vi "niFPGA 32-Bit Cast Emit Code.vi"(0 "Emit Code Info In":refnum<class "EmitCode(DiagramComponent).lvclass">, 11 "error in (no error)":errorcluster) -> (4 "Emit Code Info Out":refnum<class "EmitCode(DiagramComponent).lvclass">, 15 "error out":errorcluster)   [LabVIEW 2017]
uses:
  <vilib>/rvi/ClientSDK/Core/ModuleGeneration/ClassModGen/EmitCode(DiagramComponent)/EmitCode(DiagramComponent).lvclass
  e:/penguin/lvdist/win32/export/17.0/17.0.1f1/dist/vi.lib/rvi/ClientSDK/Core/ModuleGeneration/ClassModGen/ModGen/ModGen.lvclass
  e:/penguin/lvdist/win32/export/17.0/17.0.1f1/dist/vi.lib/rvi/ClientSDK/Core/ModuleGeneration/ClassModGen/EmitCode/EmitCode.lvclass
  <vilib>/rvi/ClientSDK/Core/ModuleGeneration/InstantiationUtility/Public/nirviInstantiatedPortSpec.ctl
  <vilib>/rvi/ClientSDK/Core/ModuleGeneration/InstantiationUtility/Public/nirviInstantiatedGenericSpec.ctl
  <vilib>/rvi/ClientSDK/Core/ModuleGeneration/ClassModGen/ModGen/ModGen.lvclass
  <vilib>/rvi/ClientSDK/Core/ModuleGeneration/ClassModGen/EmitCode/EmitCode.lvclass
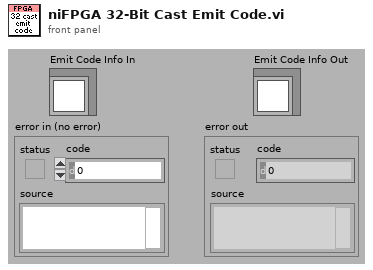
[diagram p1: front panel]
types:
  T1 = typedef "nirviInstantiatedGenericSpec.ctl" = cluster{"Static Generic Connection":string, "Generic Value If Unconnected":string, "Generic Name From Backend":string, "Pre Connection Addition":string, "Post Connection Addition":string}
  T2 = typedef "nirviInstantiatedPortSpec.ctl" = cluster{"Port Name From Backend":string, "Static Port Connection":string, "Post Signal Addition":string, "Pre Signal Addition":string, "Value If Unwired":string, "TxtToReplaceWithActualSig":string}
  T3 = cluster{"PortName":string, "PortConnection":string, "isConstant":bool, "PortWidth":i32, "Direction":enum32{"", "MOD_PORT_OUT", "MOD_PORT_IN", "MOD_PORT_INOUT"}, "Representation":enum32{"", "MOD_SIG_SIGN", "MOD_SIG_UNSIGN", "MOD_SIG_FLOAT"}, "Sig type":enum32{"", "MOD_SIG_BIT", "MOD_SIG_VECT", "MOD_SIG_ARRAY"}, "NumDimensions":i32, "DimensionSizes":i32[], "Element Width":i32, "Generic Name":string}[]
  T4 = typedef "niFpgaGeneric.ctl" = cluster{"Generic Name":string, "Port Type":string, "String Value":string, "Int Value":i64}
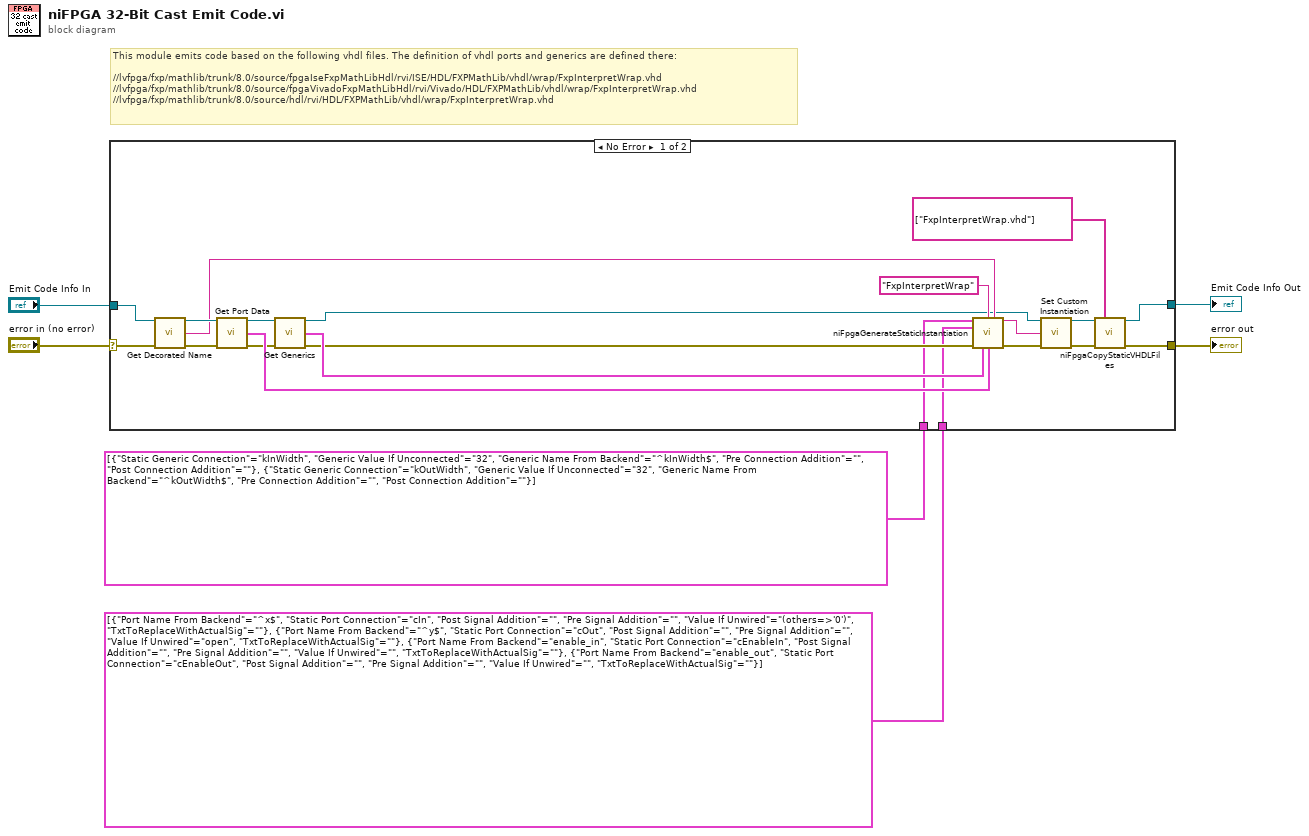
[diagram p0: block diagram]
diagram:
  # "This module emits code based on the following vhdl files. The definition of vhdl ports and generics are defined there:\n\n//lvfpga/fxp/mathlib/trunk/8.0/source/fpgaIseFxpMathLibHdl/rvi/ISE/HDL/FXPMathLib/vhdl/wrap/FxpInterpretWrap.vhd\n//lvfpga/fxp/mathlib/trunk/8.0/source/fpgaVivadoFxpMathLibHdl/rvi/Vivado/HDL/FXPMathLib/vhdl/wrap/FxpInterpretWrap.vhd\n//lvfpga/fxp/mathlib/trunk/8.0/source/hdl/rvi/HDL/FXPMathLib/vhdl/wrap/FxpInterpretWrap.vhd"
  n1 = case shown="No Error" "error in (no error)" {
    selector: "error in (no error)" -> [w16 w28]
    tunnel: "Emit Code Info In" -> [w17 w29]
    tunnel: [w11 w28] -> w5
    tunnel: [w9 w29] -> w4
    tunnel: T2[] [{"Port Name From Backend"="^x$", "Static Port Connection"="cIn", "Post Signal Addition"="", "Pre Signal Addition"="", "Value If Unwired"="(others=>'0')", "TxtToReplaceWithActualSig"=""}, {"Port Name From Backend"="^y$", "Static Port Connection"="cOut", "Post Signal Addition"="", "Pre Signal Addition"="", "Value If Unwired"="open", "TxtToReplaceWithActualSig"=""}, {"Port Name From Backend"="enable_in", "Static Port Connection"="cEnableIn", "Post Signal Addition"="", "Pre Signal Addition"="", "Value If Unwired"="", "TxtToReplaceWithActualSig"=""}, {"Port Name From Backend"="enable_out", "Static Port Connection"="cEnableOut", "Post Signal Addition"="", "Pre Signal Addition"="", "Value If Unwired"="", "TxtToReplaceWithActualSig"=""}] ("Static Ports") -> [w13 _]
    tunnel: T1[] [{"Static Generic Connection"="kInWidth", "Generic Value If Unconnected"="32", "Generic Name From Backend"="^kInWidth$", "Pre Connection Addition"="", "Post Connection Addition"=""}, {"Static Generic Connection"="kOutWidth", "Generic Value If Unconnected"="32", "Generic Name From Backend"="^kOutWidth$", "Pre Connection Addition"="", "Post Connection Addition"=""}] -> [w7 _]
    frame No Error {
      n2 = call <vilib>:"Get Decorated Name.vi"("ModGen in"=w17, "error in (no error)"=w16) -> ("ModGen out"=w24:refnum<class "EmitCode(DiagramComponent).lvclass">, "Decorated Name"=w22:string, "error out"=w23:errorcluster)  [unwired: 11 in]
      n3 = call <vilib>:"Get Port Data.vi"("CodeGenInfo(Resource) in"=w24, "error in (no error)"=w23) -> ("CodeGenInfo(Resource) out"=w19:refnum<class "EmitCode(DiagramComponent).lvclass">, "Port Data"=w26:T3, "error out"=w20:errorcluster)  [unwired: 11 in]
      n4 = call <vilib>:"Get Generics.vi"("ModGenInfo in"=w19, "error in (no error)"=w20) -> ("ModGenInfo out"=w15:refnum<class "EmitCode(DiagramComponent).lvclass">, "Generics"=w18:T4[], "error out"=w14:errorcluster)  [unwired: 11 in]
      n5 = call <vilib>:"niFpgaGenerateStaticInstantiation.vi"("Static Generics"=w7, "Entity Name"="FxpInterpretWrap", "Decorated Name Used For Instance Name"=w22, "Static Ports"=w13, "error in (no error)"=w14, "Generic Data From LabVIEW"=w18, "Port Data From LabVIEW"=w26) -> ("Instantiation"=w21:string, "error out"=w27:errorcluster)  [unwired: 1 in, 6 out]
      n6 = call <vilib>:"Set Custom Instantiation.vi"("CodeGenInfo(Resource) in"=w15, "instantiation"=w21, "error in (no error)"=w27) -> ("CodeGenInfo(Resource) out"=w10:refnum<class "EmitCode(DiagramComponent).lvclass">, "error out"=w12:errorcluster)  [unwired: 11 in]
      n7 = call <vilib>:"niFpgaCopyStaticVHDLFiles.vi"("CodeGenInfo(Resource) in"=w10, "static VHDL file names"=string[] ["FxpInterpretWrap.vhd"], "error in"=w12) -> ("CodeGenInfo(Resource) out"=w9:refnum<class "EmitCode(DiagramComponent).lvclass">, "error out"=w11:errorcluster)  [unwired: 11 out]
    }
    frame Error {
    }
  }
  "Emit Code Info Out" <- w4
  "error out" <- w5
